vi "Create Log File.vi"(10 "Mode":T1(ring), 11 "string":string) -> (0 "File Write Error":errorcluster, 3 "Byte Stream File out":refnum<file>)   [LabVIEW 2020]
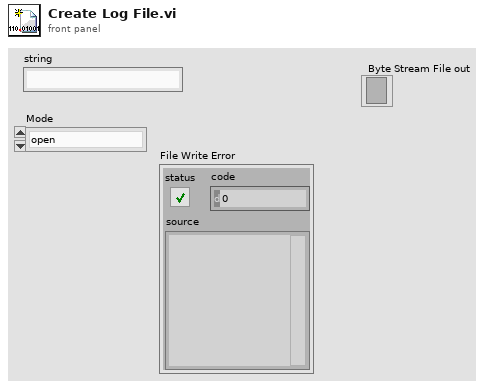
[diagram p1: front panel]
types:
  T1 = enum16{"open", "replace", "create", "open or create", "replace or create", "replace or create with confirmation"}
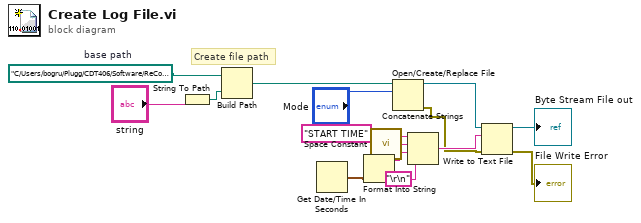
[diagram p0: block diagram]
diagram:
  w15 = path "C:/Users/bogru/Plugg/CDT406/Software/ReCog/Recog-system/Logfiles"  # base path
  # "Create file path"
  n1 = String To Path(string="string") -> (path=w14:path)
  n2 = Build Path(base path=w15, name or relative path=w14) -> (appended path=w13:path)
  n3 = Get Date/Time In Seconds() -> (seconds since 1Jan1904=w7:timestamp)
  n4 = Format Into String(w7) -> (resulting string=w4:string)  [unwired: 3 in, 1 out]
  n5 = call <vilib>:"Space Constant.vi"() -> ("String"=w5:string)
  n6 = Open/Create/Replace File(file path (use dialog)=w13, operation (0:open)="Mode") -> (refnum out=w12:refnum<file>, error out=w9:errorcluster)  [unwired: 4 in, 1 out]
  n7 = Concatenate Strings("START TIME", w5, w4, "\r\n") -> (w11:string)
  n8 = Write to Text File(file (use dialog)=w12, text=w11, error in=w9) -> (refnum out=→"Byte Stream File out":refnum<file>, error out=→"File Write Error":errorcluster)  [unwired: 1 in, 1 out]
